vi "Set Z Scale Marker Values.vi"(8 "error in (no error)":errorcluster, 10 "Z Scale.Marker Values[]":cluster{dbl, u32}[](array[cluster]), 11 "Base Graph in":refnum<class "Base Graph.lvclass">) -> (0 "error out":errorcluster, 3 "Base Graph out":refnum<class "Base Graph.lvclass">)   [LabVIEW 2023, in "Base Graph.lvclass"]
uses:
  Base Graph.lvclass
  Base Graph.lvclass/Base Graph.ctl
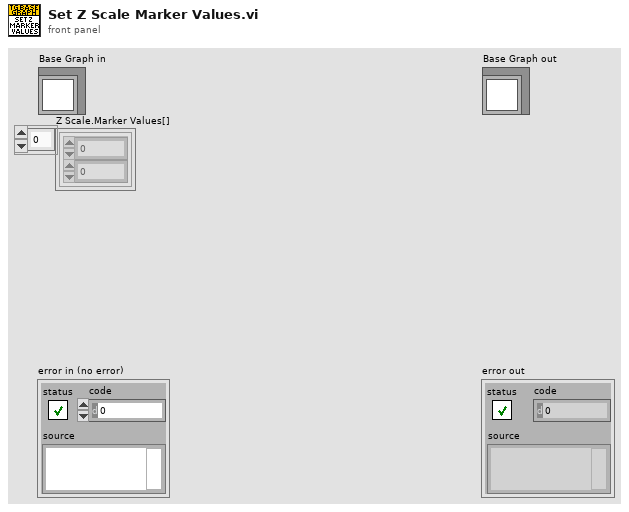
[diagram p1: front panel]
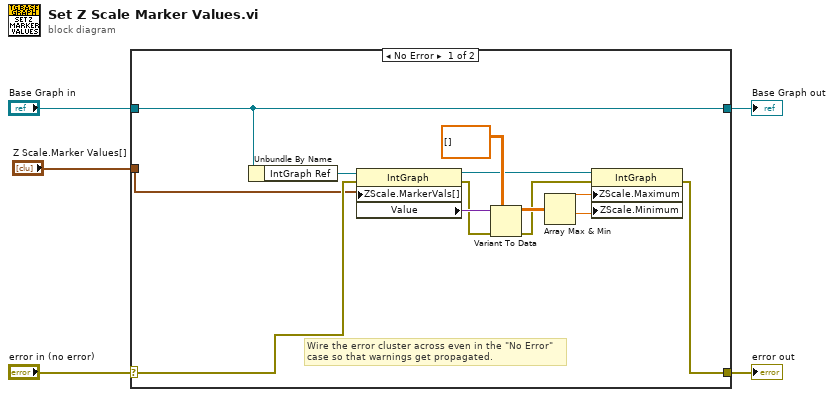
[diagram p0: block diagram]
diagram:
  n1 = case shown="No Error" "error in (no error)" {
    selector: "error in (no error)" -> [w16 w20]
    tunnel: [w8 w20] -> w4
    tunnel: [w18 w19] -> w2
    tunnel: "Base Graph in" -> [w18 w19]
    tunnel: "Z Scale.Marker Values[]" -> [w15 _]
    frame No Error {
      # "Wire the error cluster across even in the \"No Error\"\ncase so that warnings get propagated."
      n2 = Unbundle By Name(w18) -> ("IntGraph Ref"=w17:refnum<vi>)
      n3 = property class="IntGraph"(reference=w17, error in=w16, "ZScale.MarkerVals[]"=w15) -> (reference out=w10:refnum<vi>, error out=w13:errorcluster, "Value"=w14:variant)
      n4 = Variant To Data(error in=w13, type=dbl[][] [], Variant=w14) -> (data=w11:dbl[][], error out=w9:errorcluster)
      n5 = Array Max & Min(array=w11) -> (max value=w7:dbl, min value=w6:dbl)  [unwired: 2 out]
      n6 = property class="IntGraph"(reference=w10, error in=w9, "ZScale.Maximum"=w7, "ZScale.Minimum"=w6) -> (error out=w8:errorcluster)  [unwired: 1 out]
    }
    frame Error {
    }
  }
  "error out" <- w4
  "Base Graph out" <- w2
